vi "get remaining time budget.vi"(8 "error in":errorcluster, 10 "dt":u32=1, 11 "timing source in":refnum<class "absolute usec timing source.lvclass">) -> (0 "error out":errorcluster, 2 "budget (ns)":u64, 3 "timing source out":refnum<class "absolute usec timing source.lvclass">)   [LabVIEW 2013, in "absolute usec timing source.lvclass"]
uses:
  absolute usec timing source.lvclass
  absolute usec timing source.lvclass/absolute usec timing source.ctl
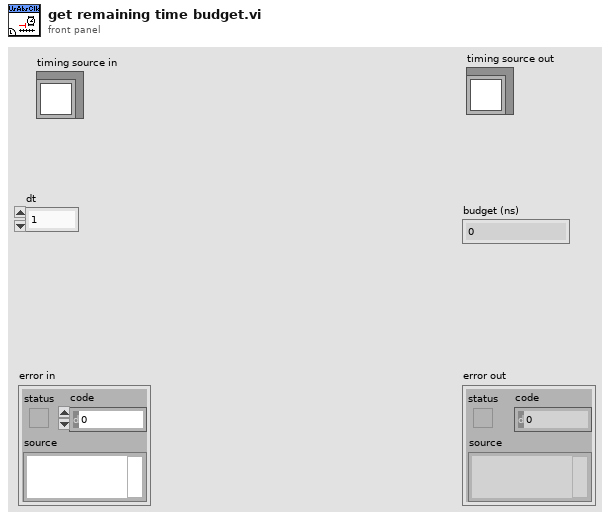
[diagram p1: front panel]
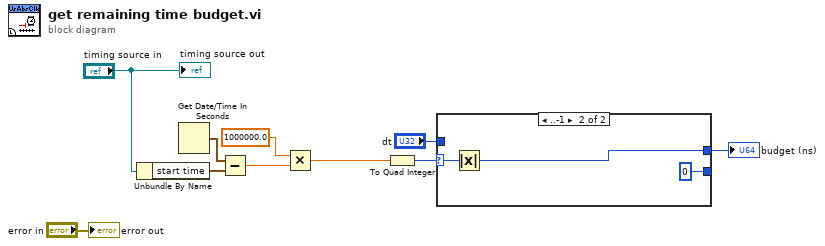
[diagram p0: block diagram]
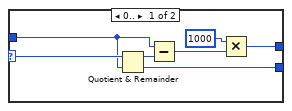
[diagram p2: hidden frame]
diagram:
  n1 = Unbundle By Name("timing source in") -> ("start time"=w9:timestamp)
  n2 = Get Date/Time In Seconds() -> (seconds since 1Jan1904=w8:timestamp)
  n3 = Subtract(x=w8, y=w9) -> (x-y=w7:dbl)
  n4 = Multiply(x=1000000.0, y=w7) -> (x*y=w5:dbl)
  n5 = To Quad Integer(1:w5) -> (0:w4:i64)
  n6 = case shown="..-1" w4 {
    selector: w4 -> [w17 w20]
    tunnel: "dt" -> [w15 _]
    tunnel: [w12 w19] -> w2
    tunnel: [w13 i64 0] -> _
    frame 0.. {
      n7 = Quotient & Remainder(x=w17, y=w15) -> (x-y*floor(x/y)=w16:i64, floor(x/y)=w13:i64)
      n8 = Subtract(x=w15, y=w16) -> (x-y=w14:i64)
      n9 = Multiply(x=i64 1000, y=w14) -> (x*y=w12:i64)
    }
    frame ..-1 {
      n10 = Absolute Value(x=w20) -> (abs(x)=w19:i64)
    }
  }
  "budget (ns)" <- w2
  "error out" <- "error in"
  "timing source out" <- "timing source in"
